vi "FM_td.vi"() -> ()   [LabVIEW 2013]
uses:
  <vilib>/sound2/lvsound2.llb/Sound File Info (path).vi
  <vilib>/sound2/lvsound2.llb/Sound File Read Open.vi
  <vilib>/sound2/lvsound2.llb/Sound File Read (DBL).vi
  <vilib>/Waveform/WDTOps.llb/WDT Get Waveform Subset DBL.vi
  <vilib>/express/express analysis/Spectral/Block/exnSpectralBlock spectral measurements RMS poly.vi
  <vilib>/express/express analysis/Spectral/Block/exnSpectralBlock spectral measurements RMS DDT.vi
  <vilib>/express/express analysis/Spectral/XNode/ExpressSpectralMeasurementsBlockNode.xnode
panel:
  in  "WAV Sample Rate 2":dbl=44100.0 caption="dt"
  in  "LPF Cut-Off 2":dbl=3000.0 caption="Lower Cut-Off"
  in  "SNR 2":dbl(slide)=30.0 caption="Standard deviation" scale=-20.0..50.0
  in  "Carrier Amp. 2":dbl=1.0 caption="Amplitude"
  in  "k_f 2":dbl(slide)=50000.0 scale=0.0..50000.0
  in  "Carrier Freq. 2":dbl=100000.0 caption="Frequency"
  out "Baseband 2":dynamicdata(graph)
  in  "Modulated Signal Source 2":enum32{"Single Tone", "From File"}(tab)
  in  "ST Frequency 2":dbl=2000.0 caption="Frequency"
  in  "ST Amplitude 2":dbl=1.0 caption="Amplitude"
  in  "Resample Rate 2":dbl=1000000.0 format="%#_6f"
  in  "Duration 2":dbl=44100.0
  in  "WAV Path 2":path=path "E:/07/0409/mozart.wav" caption="Path"
  in  "Normalized Peak Amplitude 2":dbl=1.0 caption="Peak Amplitude"
  in  "Modulated Signal Source 1":enum32{"Single Tone", "From File"}(tab)
  in  "ST Frequency 1":dbl=2000.0 caption="Frequency"
  in  "ST Amplitude 1":dbl=1.0 caption="Amplitude"
  in  "Resample Rate 1":dbl=1000000.0 format="%#_6f"
  in  "Duration 1":dbl=44100.0
  in  "WAV Path 1":path=path "E:/07/0409/mozart.wav" caption="Path"
  in  "Normalized Peak Amplitude 1":dbl=1.0 caption="Peak Amplitude"
  in  "WAV Sample Rate 1":dbl=44100.0 caption="dt"
  in  "LPF Cut-Off 1":dbl=3000.0 caption="Lower Cut-Off"
  in  "SNR 1":dbl(slide)=30.0 caption="Standard deviation" scale=-20.0..50.0
  out "Recovered Signal 1":dynamicdata(graph)
  out "Baseband 1":dynamicdata(graph)
  out "FM FFT":dynamicdata(graph)
  out "FM Wave":dynamicdata(graph)
  in  "Carrier Amp. 1":dbl=1.0 caption="Amplitude"
  in  "stop":bool
  in  "k_f 1":dbl(slide)=50000.0 scale=0.0..50000.0
  in  "Carrier Freq. 1":dbl=100000.0 caption="Frequency"
  # "Frequency Modulation"
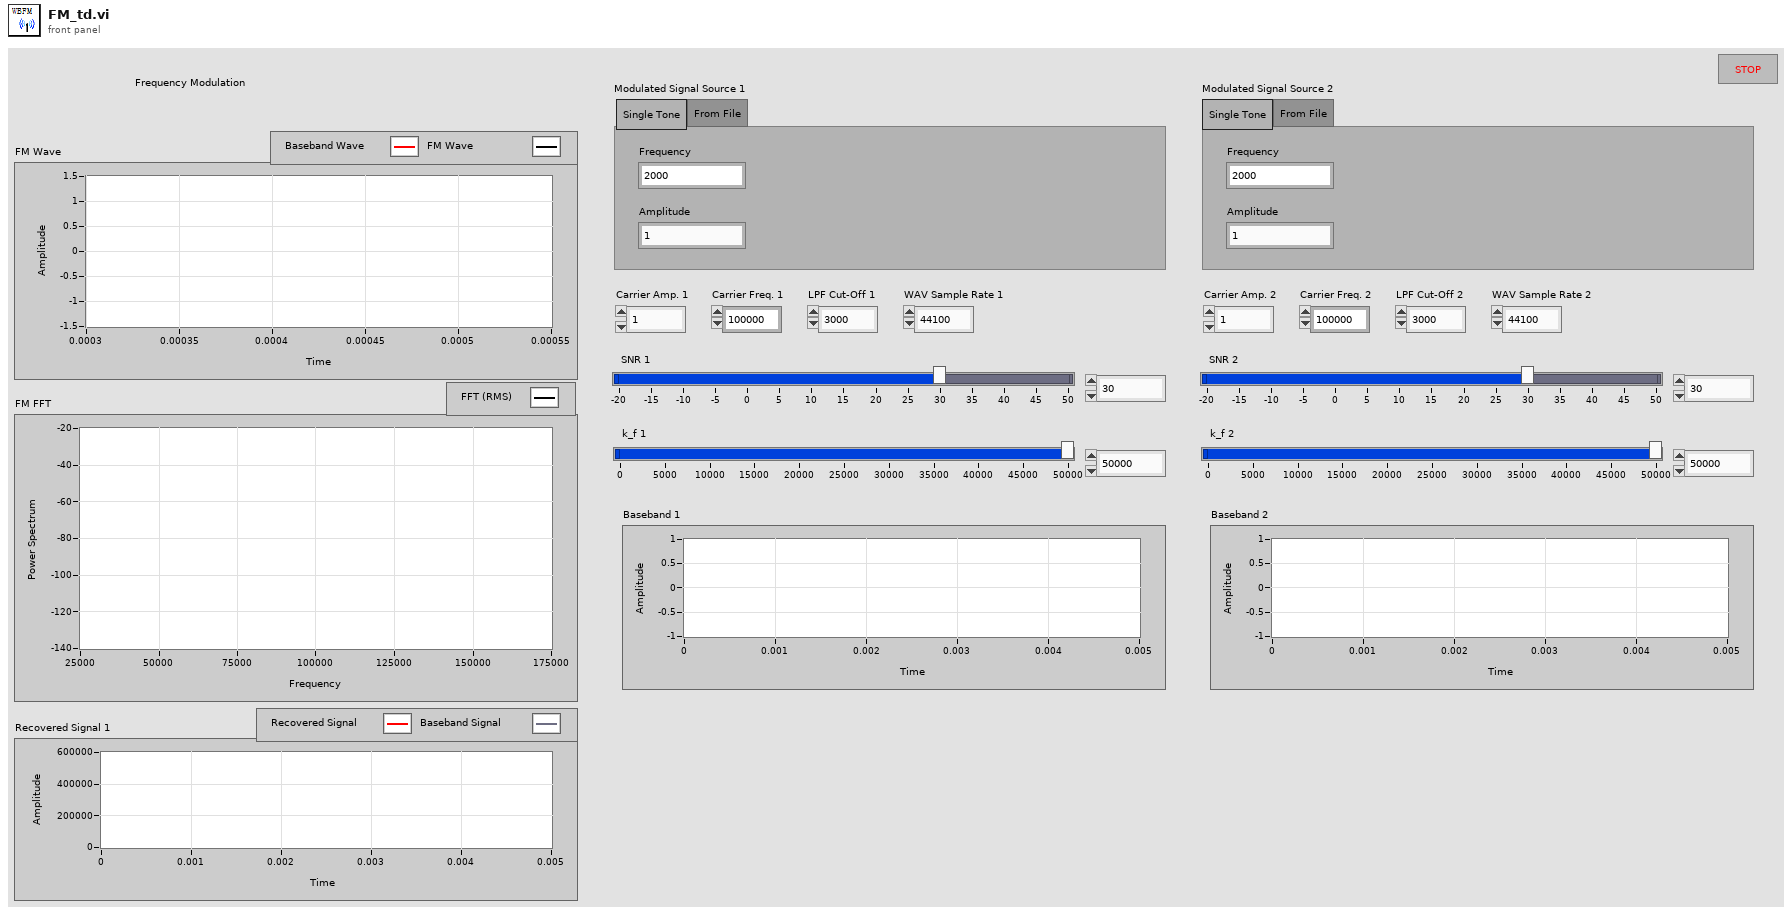
[diagram p1: front panel]
types:
  T1 = cluster{"averaging mode":u16, "weighting mode":u16, "number of averages":u32}
  T2 = cluster{"dB On (F)":bool, "unwrap phase (F)":bool, "convert to degree (F)":bool}
  T3 = typedef "Sound File Refnum.ctl" = refnum<file>
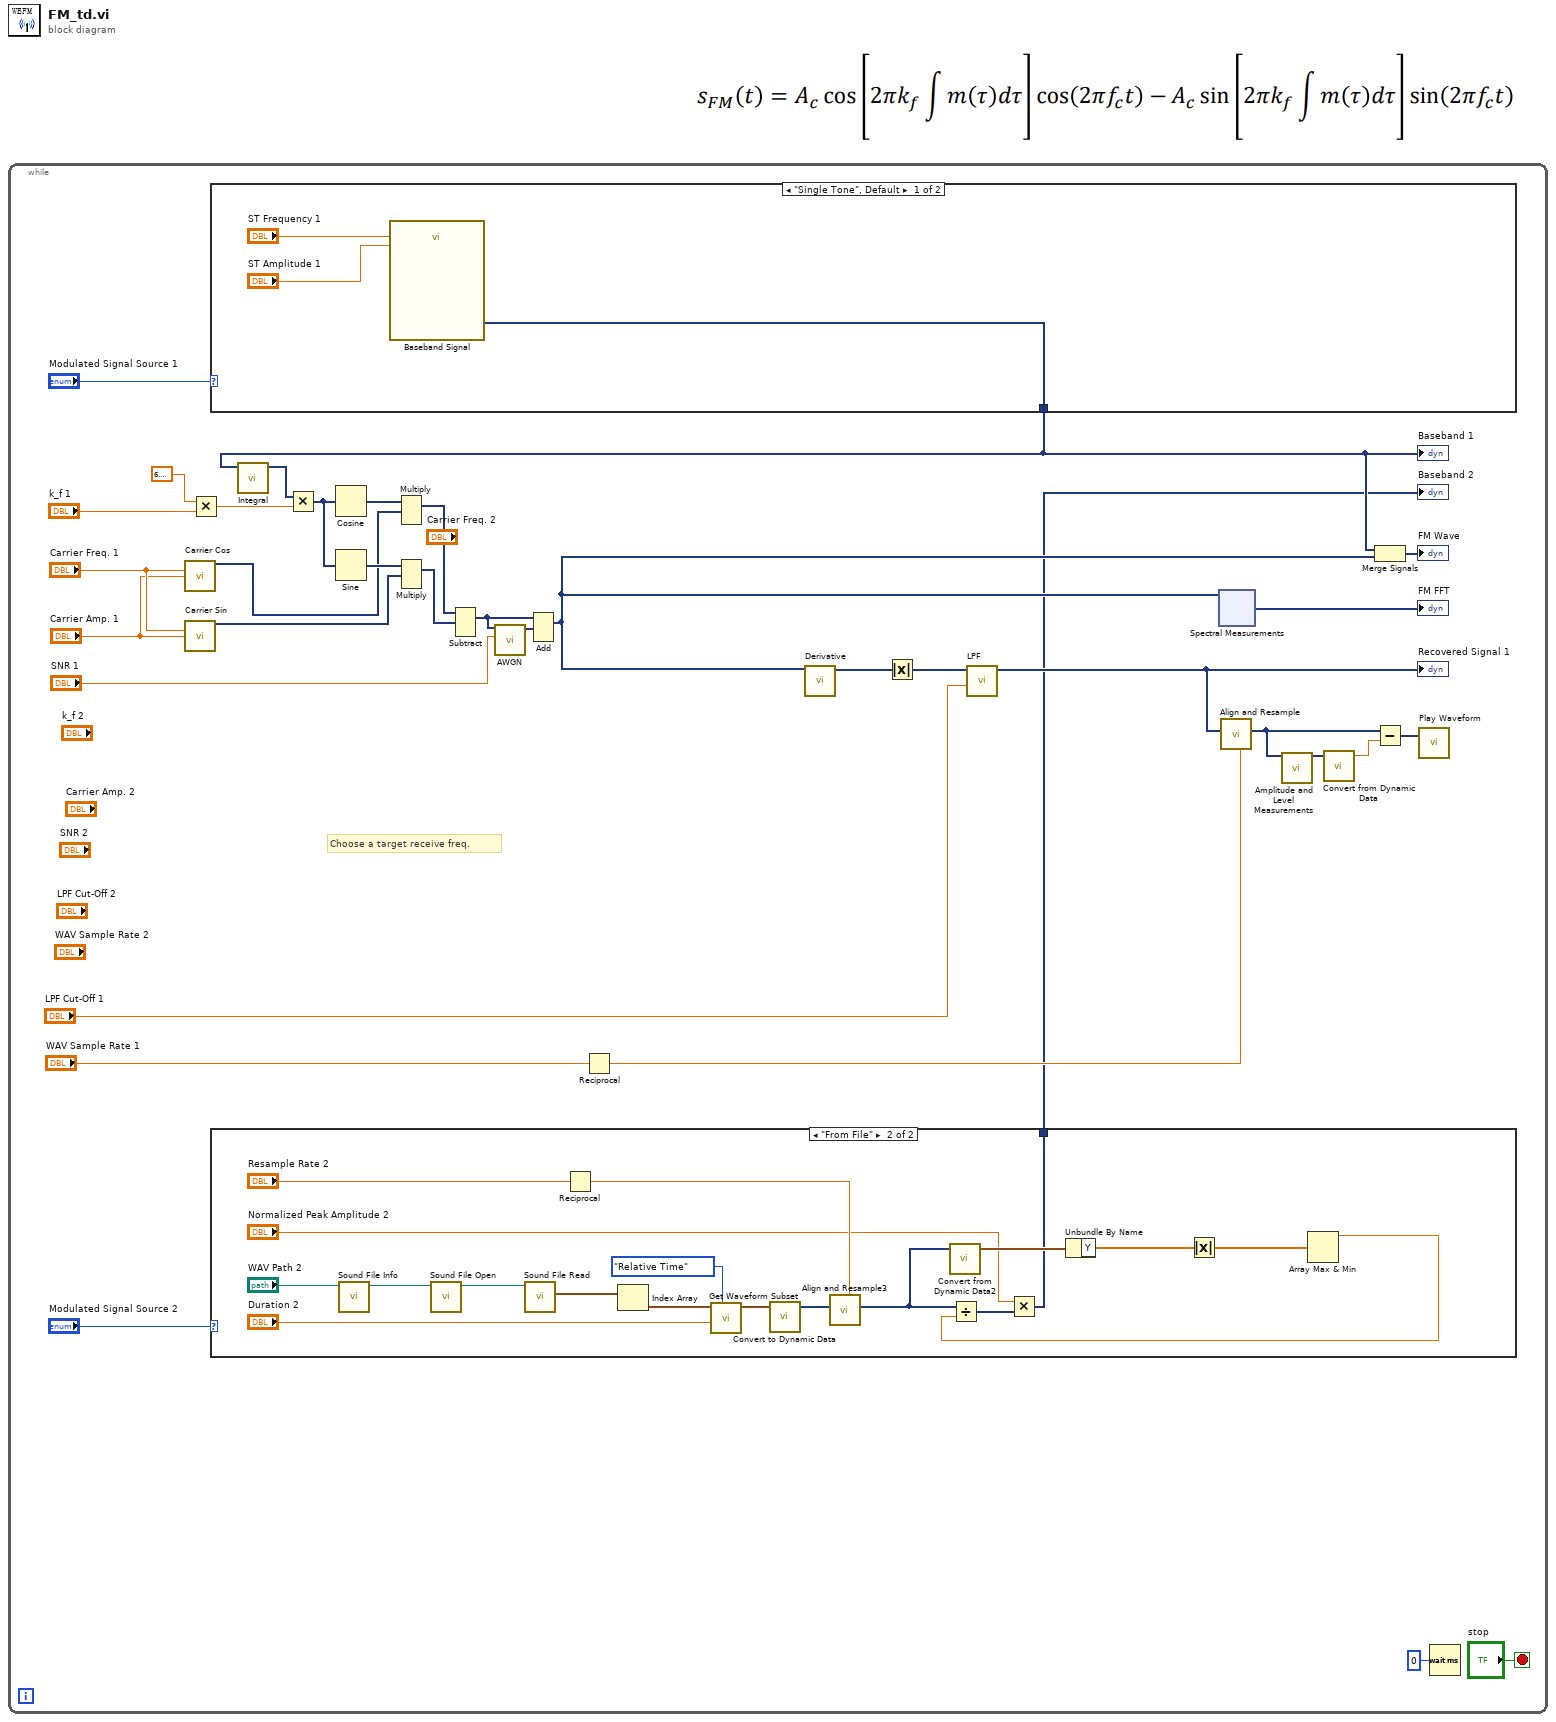
[diagram p0: block diagram]
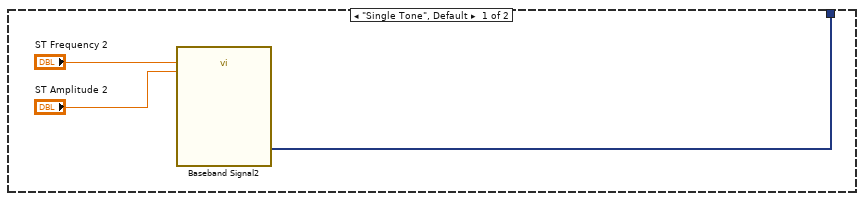
[diagram p2: hidden frame]
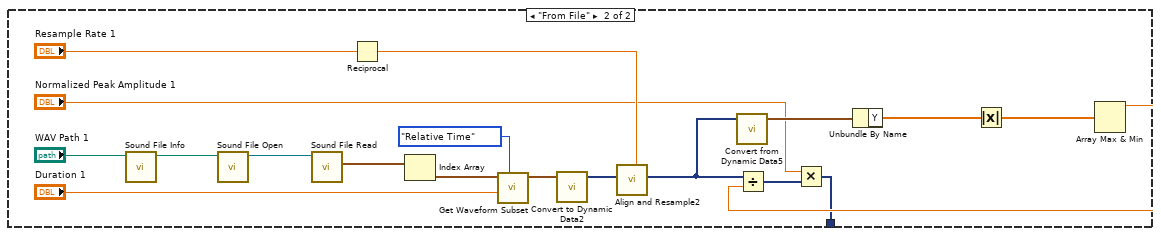
[diagram p3: hidden frame]
diagram:
  n1 = while {
    stop <- "stop" stop-if-true
    # "Choose a target receive freq."
    n2 = call "Carrier Cos"("Frequency"="Carrier Freq. 1", "Amplitude"="Carrier Amp. 1") -> ("Sine"=w15:dynamicdata)  [unwired: 12 in, 1 out]
    n3 = call "Carrier Sin"("Frequency"="Carrier Freq. 1", "Amplitude"="Carrier Amp. 1") -> ("Sine"=w14:dynamicdata)  [unwired: 12 in, 1 out]
    n4 = Multiply(x=6.283185307179586, y="k_f 1") -> (x*y=w8:dbl)
    n5 = case shown="\"Single Tone\", Default" "Modulated Signal Source 1" {
      tunnel: [w58 w62] -> w9
      frame "Single Tone", Default {
        n6 = call "Baseband Signal"("Frequency"="ST Frequency 1", "Amplitude"="ST Amplitude 1") -> ("Sine"=w58:dynamicdata)  [unwired: 12 in, 1 out]
      }
      frame "From File" {
        n7 = call-poly <vilib>:"Sound File Info.vi"("path"="WAV Path 1") -> ("path out"=w77:path)  [unwired: 7 in, 3 out]
        n8 = call-poly <vilib>:"Sound File Open.vi"("path"=w77) -> ("sound file refnum"=w79:T3)  [unwired: 9 in, 1 out]
        n9 = call-poly <vilib>:"Sound File Read.vi"("sound file refnum"=w79) -> ("data"=w74:waveform(dbl)[])  [unwired: 6 in, 4 out]
        n10 = Reciprocal(x="Resample Rate 1") -> (1/x=w70:dbl)
        n11 = Index Array(array=w74) -> (element=w75:waveform(dbl))  [unwired: 1 in]
        n12 = call-poly <vilib>:"Get Waveform Subset.vi"("start/duration format"=enum16{"Relative Time"}."Relative Time", "duration"="Duration 1", "waveform in"=w75) -> ("waveform out"=w69:waveform(dbl))  [unwired: 3 in, 3 out]
        n13 = call "Convert to Dynamic Data2"("Waveform"=w69) -> ("Dynamic Data Type"=w64:dynamicdata)  [unwired: 3 in]
        n14 = call "Align and Resample2"("dt"=w70, "Signals"=w64) -> ("Resampled Signals"=w65:dynamicdata)  [unwired: 7 in, 2 out]
        n15 = call "Convert from Dynamic Data5"("Dynamic Data Type"=w65) -> ("Waveform"=w72:waveform(dbl))  [unwired: 3 in]
        n16 = Unbundle By Name(w72) -> ("Y"=w66:dbl[])
        n17 = Absolute Value(x=w66) -> (abs(x)=w68:dbl[])
        n18 = Array Max & Min(array=w68) -> (max value=w67:dbl)  [unwired: 3 out]
        n19 = Divide(x=w65, y=w67) -> (x/y=w63:dynamicdata)
        n20 = Multiply(x="Normalized Peak Amplitude 1", y=w63) -> (x*y=w62:dynamicdata)
      }
    }
    "Baseband 1" <- w9
    n21 = case shown="\"From File\"" "Modulated Signal Source 2" {
      tunnel: [w36 w40] -> w1
      frame "Single Tone", Default {
        n22 = call "Baseband Signal2"("Frequency"="ST Frequency 2", "Amplitude"="ST Amplitude 2") -> ("Sine"=w36:dynamicdata)  [unwired: 12 in, 1 out]
      }
      frame "From File" {
        n23 = call-poly <vilib>:"Sound File Info.vi"("path"="WAV Path 2") -> ("path out"=w55:path)  [unwired: 7 in, 3 out]
        n24 = call-poly <vilib>:"Sound File Open.vi"("path"=w55) -> ("sound file refnum"=w57:T3)  [unwired: 9 in, 1 out]
        n25 = call-poly <vilib>:"Sound File Read.vi"("sound file refnum"=w57) -> ("data"=w52:waveform(dbl)[])  [unwired: 6 in, 4 out]
        n26 = Reciprocal(x="Resample Rate 2") -> (1/x=w48:dbl)
        n27 = Index Array(array=w52) -> (element=w53:waveform(dbl))  [unwired: 1 in]
        n28 = call-poly <vilib>:"Get Waveform Subset.vi"("start/duration format"=enum16{"Relative Time"}."Relative Time", "duration"="Duration 2", "waveform in"=w53) -> ("waveform out"=w47:waveform(dbl))  [unwired: 3 in, 3 out]
        n29 = call "Convert to Dynamic Data"("Waveform"=w47) -> ("Dynamic Data Type"=w42:dynamicdata)  [unwired: 3 in]
        n30 = call "Align and Resample3"("dt"=w48, "Signals"=w42) -> ("Resampled Signals"=w43:dynamicdata)  [unwired: 7 in, 2 out]
        n31 = call "Convert from Dynamic Data2"("Dynamic Data Type"=w43) -> ("Waveform"=w50:waveform(dbl))  [unwired: 3 in]
        n32 = Unbundle By Name(w50) -> ("Y"=w44:dbl[])
        n33 = Absolute Value(x=w44) -> (abs(x)=w46:dbl[])
        n34 = Array Max & Min(array=w46) -> (max value=w45:dbl)  [unwired: 3 out]
        n35 = Divide(x=w43, y=w45) -> (x/y=w41:dynamicdata)
        n36 = Multiply(x="Normalized Peak Amplitude 2", y=w41) -> (x*y=w40:dynamicdata)
      }
    }
    "Baseband 2" <- w1
    n37 = call "Integral"("Signals"=w9) -> ("Result"=w10:dynamicdata)  [unwired: 5 in, 1 out]
    n38 = Multiply(x=w10, y=w8) -> (x*y=w19:dynamicdata)
    n39 = Cosine(x=w19) -> (cos(x)=w21:dynamicdata)
    n40 = Sine(x=w19) -> (sin(x)=w20:dynamicdata)
    n41 = Multiply(1:w15, 2:w21) -> (0:w17:dynamicdata)  [unwired: 1 in, 1 out]
    n42 = Multiply(1:w14, 2:w20) -> (0:w16:dynamicdata)  [unwired: 1 in, 1 out]
    n43 = Subtract(1:w16, 2:w17) -> (0:w18:dynamicdata)  [unwired: 1 in, 1 out]
    n44 = call "AWGN.vi"("SNR (dB)"="SNR 1", "Dynamic Data"=w18) -> ("DC with Gaussian Noise"=w25:dynamicdata)  [unwired: 9 in]
    n45 = Add(1:w25, 2:w18) -> (0:w7:dynamicdata)  [unwired: 1 in, 1 out]
    n46 = Reciprocal(x="WAV Sample Rate 1") -> (1/x=w22:dbl)
    n47 = call "Derivative"("Signals"=w7) -> ("Result"=w6:dynamicdata)  [unwired: 5 in, 1 out]
    n48 = Absolute Value(x=w6) -> (abs(x)=w5:dynamicdata)
    n49 = call "LPF"("Lower Cut-Off"="LPF Cut-Off 1", "Signal"=w5) -> ("Filtered Signal"=w3:dynamicdata)  [unwired: 8 in, 1 out]
    "Recovered Signal 1" <- w3
    n50 = xnode ("Spectral Measurements")("Signals"=w7) -> ("FFT - (RMS)"=→"FM FFT":dynamicdata)  [unwired: 1 in, 2 out]
    n51 = call "Align and Resample"("dt"=w22, "Signals"=w3) -> ("Resampled Signals"=w12:dynamicdata)  [unwired: 7 in, 2 out]
    n52 = call "Amplitude and Level Measurements"("Signals"=w12) -> ("Mean (DC)"=w31:dynamicdata)  [unwired: 13 in, 1 out]
    n53 = call "Convert from Dynamic Data"("Dynamic Data Type"=w31) -> ("Scalar"=w32:dbl)  [unwired: 3 in]
    n54 = Merge Signals(w9, w7) -> (→"FM Wave":dynamicdata)
    n55 = Subtract(x=w12, y=w32) -> (x-y=w13:dynamicdata)
    n56 = call "Play Waveform"("Data"=w13) -> ()  [unwired: 18 in, 1 out]
    n57 = Wait (ms)(milliseconds to wait=u32 0) -> ()  [unwired: 1 out]
  }
